vi "needBreak.vi"(0 "Game in":refnum<class "Game.lvclass">, 1 "v_sample":dbl, 3 "delta":dbl, 5 "Robot":refnum<class "Robot.lvclass">, 9 "dest":dbl[](array[numeric]) format="%#_13g", 11 "error in (no error)":errorcluster, 12 "firstCall":bool=TRUE, 14 "desired_vel":dbl format="%#_13g") -> (4 "Game out":refnum<class "Game.lvclass">, 6 "needBreak":bool=TRUE, 8 "velocityBreakState":T1, 10 "vel":dbl, 15 "error out":errorcluster)   [LabVIEW 2020, in "Game.lvclass"]
uses:
  Game.lvclass
  Robot_class/Robot.lvclass
  Controls/velocityBreakState.ctl
  Object_class/Object.lvclass/Object.ctl
  <vilib>/Analysis/_algsub.llb/Real Vector Norm.vi
  Object_class/Read x.vi
  Object_class/Read y.vi
  Utilities_class/Utilities.lvclass
  <vilib>/Analysis/NI_AALPro.lvlib
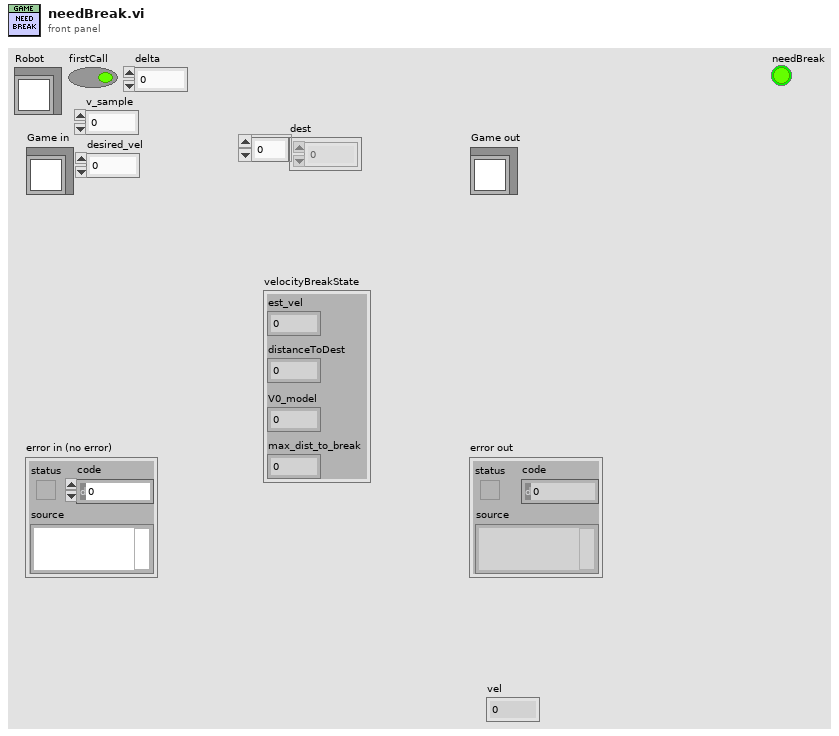
[diagram p1: front panel]
types:
  T1 = typedef "velocityBreakState.ctl" = cluster{"est_vel":dbl, "distanceToDest":dbl, "V0_model":dbl, "max_dist_to_break":dbl}
  T2 = typedef "RobotModel.ctl" = cluster{"V0":dbl, "Vf":dbl, "Dist":dbl, "dt":dbl, "P1":dbl[], "P2":dbl[], "V_sent":dbl}
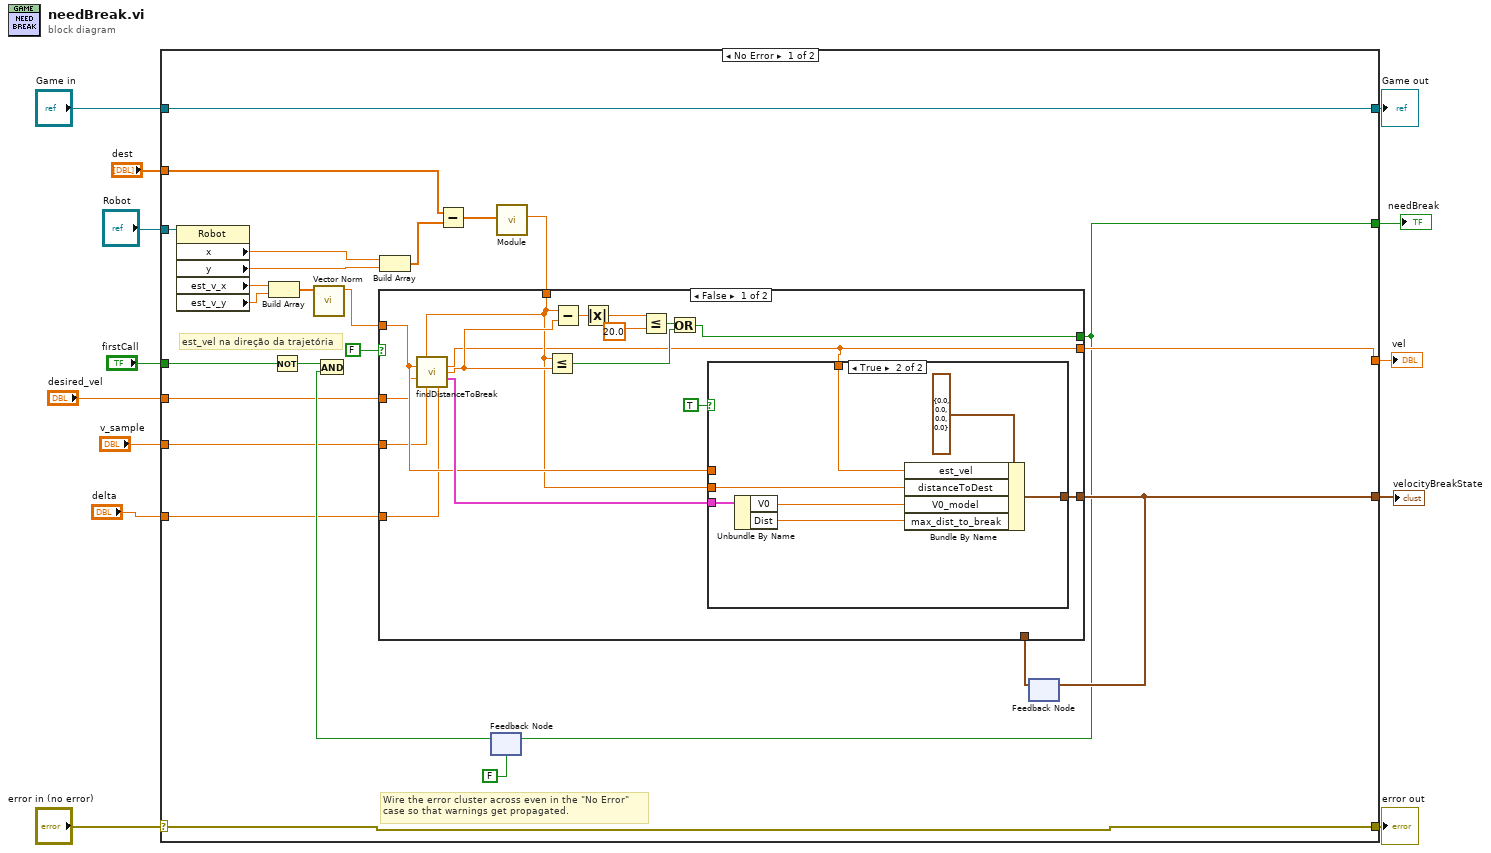
[diagram p0: block diagram]
diagram:
  n1 = case shown="No Error" "error in (no error)" {
    selector: "error in (no error)" -> [w37 w65]
    tunnel: [w37 w65] -> w12
    tunnel: [w38 w64] -> w10
    tunnel: "Game in" -> [w38 w64]
    tunnel: "Robot" -> [w36 _]
    tunnel: "dest" -> [w33 _]
    tunnel: [w14 _] -> w7
    tunnel: "firstCall" -> [w28 _]
    tunnel: [w27 _] -> w5
    tunnel: "v_sample" -> [w25 _]
    tunnel: "delta" -> [w24 _]
    tunnel: "desired_vel" -> [w23 _]
    tunnel: [w15 _] -> w1
    frame No Error {
      # "est_vel na direção da trajetória"
      # "Wire the error cluster across even in the \"No Error\"\ncase so that warnings get propagated."
      n2 = property class="Robot"(reference=w36) -> ("x"=w32:dbl, "y"=w35:dbl, "est_v_x"=w20:dbl, "est_v_y"=w19:dbl)  [unwired: 1 in, 2 out]
      n3 = Build Array(w20, w19) -> (w18:dbl[])
      n4 = Not(x=w28) -> (.not. x?=w29:bool)
      n5 = call-poly <vilib>:"Vector Norm.vi"("Input Vector"=w18) -> ("norm"=w17:dbl)  [unwired: 9 in, 1 out]
      n6 = Build Array(w32, w35) -> (w34:dbl[])
      n7 = Subtract(x=w33, y=w34) -> (x-y=w22:dbl[])
      n8 = feedback #1(FALSE) -> (w30:bool)
      n9 = And(x=w29, y=w30) -> ()  [unwired: 1 out]
      n10 = call "Module.vi"("2D vector"=w22) -> ("Modulo"=w21:dbl)  [unwired: 8 in, 2 out]
      n11 = feedback #2() -> (w26:T1)  [unwired: 1 in]
      n12 = case shown="False" FALSE {
        selector: FALSE -> [_ w63]
        tunnel: w17 -> [w47 _]
        tunnel: w21 -> [w40 _]
        tunnel: [w46 w63] -> w14
        tunnel: [w49 w62] -> w27
        tunnel: w26 -> [_ w62]
        tunnel: w25 -> [w45 _]
        tunnel: w24 -> [w44 _]
        tunnel: w23 -> [w43 _]
        tunnel: [w39 _] -> w15
        frame False {
          n13 = call "findDistanceToBreak.vi"("dist_robot_target"=w40, "est_vel"=w47, "desired_vel"=w43, "v_sample"=w45, "delta"=w44) -> ("vel"=w39:dbl, "DistanceToBreak"=w41:dbl, "Robot Model"=w48:T2)  [unwired: 6 in, 2 out]
          n14 = Less Or Equal?(x=w40, y=w41) -> (x <= y?=w50:bool)
          n15 = Subtract(x=w40, y=w41) -> (x-y=w54:dbl)
          n16 = Absolute Value(x=w54) -> (abs(x)=w52:dbl)
          n17 = Less Or Equal?(x=w52, y=20.0) -> (x <= y?=w51:bool)
          n18 = Or(x=w51, y=w50) -> (x .or. y?=w46:bool)
          n19 = case shown="True" TRUE {
            tunnel: [_ w60] -> w49
            tunnel: w47 -> [_ _]
            tunnel: w40 -> [_ w59]
            tunnel: w48 -> [_ w58]
            tunnel: w39 -> [_ w55]
            frame False {
            }
            frame True {
              n20 = Unbundle By Name(w58) -> ("V0"=w57:dbl, "Dist"=w56:dbl)
              n21 = Bundle By Name(cluster=T1 {"est_vel"=0.0, "distanceToDest"=0.0, "V0_model"=0.0, "max_dist_to_break"=0.0} ("velocityBreakState 2"), "est_vel"=w55, "distanceToDest"=w59, "V0_model"=w57, "max_dist_to_break"=w56) -> (w60:T1)
            }
          }
        }
        frame True {
        }
      }
      n22 = feedback-in #1(w14) -> ()
      n23 = feedback-in #2(w27) -> ()
    }
    frame Error {
    }
  }
  "error out" <- w12
  "Game out" <- w10
  "needBreak" <- w7
  "velocityBreakState" <- w5
  "vel" <- w1
